vi "FixHiddenCharacters.vi"(11 "String in":string) -> (3 "String out":string)   [LabVIEW 2020]
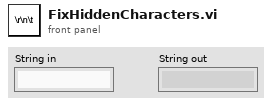
[diagram p1: front panel]
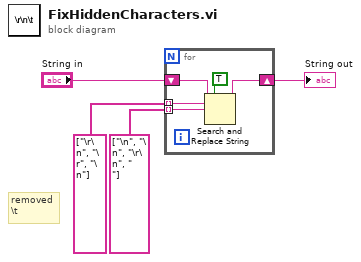
[diagram p0: block diagram]
diagram:
  # "removed\n\\t"
  n1 = for {
    tunnel: string[] ["\r\n", "\r", "\n"] -> [w7] mode=indexing
    tunnel: string[] ["\n", "\n", "\r\n", "    "] -> [w6] mode=indexing
    shift-right: [w5] -> w4
    shift-left: "String in" -> [w9]
    n2 = Search and Replace String(replace all?=TRUE ("replace all? (F)"), input string=w9, search string=w7, replace string=w6) -> (result string=w5:string)  [unwired: 4 in, 3 out]
  }
  "String out" <- w4
